vi "week7.vi"() -> ()   [LabVIEW 2014]
panel:
  out "error out 2":errorcluster caption="error out"
  in  "Digitalizing parameters":T1
  out "FFT":cluster{"f0":dbl, "df":dbl, "magnitude":dbl[]}(graph)
  out "Waveform Graph":dbl[](graph)
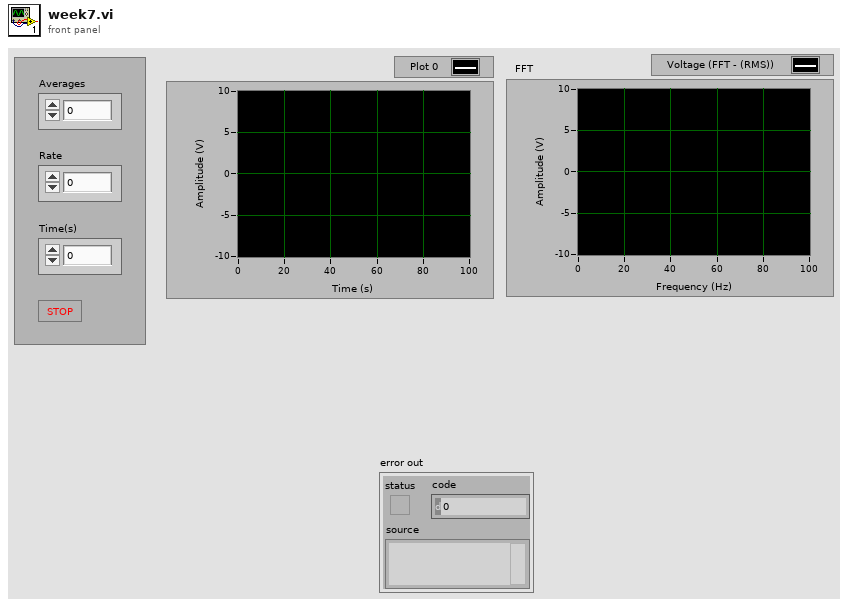
[diagram p1: front panel]
types:
  T1 = cluster{"Averages":dbl, "Rate":dbl, "Time(s)":dbl, "stop":bool}
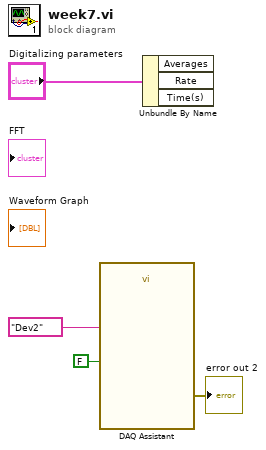
[diagram p0: block diagram]
diagram:
  n1 = call "DAQ Assistant"("stop (T)"=FALSE, "device name"=tag "Dev2") -> ("error out"=→"error out 2":errorcluster)  [unwired: 16 in, 1 out]
  n2 = Unbundle By Name("Digitalizing parameters") -> ()  [unwired: 3 out]
